vi "FEED_Check_For_indicator.vi"(7 "CURRENT PLAN":refnum<vi>, 8 "error in (no error)":errorcluster) -> (0 "error out":errorcluster)   [LabVIEW 2017]
panel:
  in  "String":string
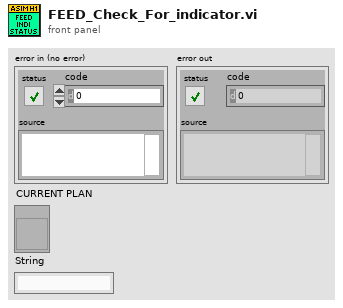
[diagram p1: front panel]
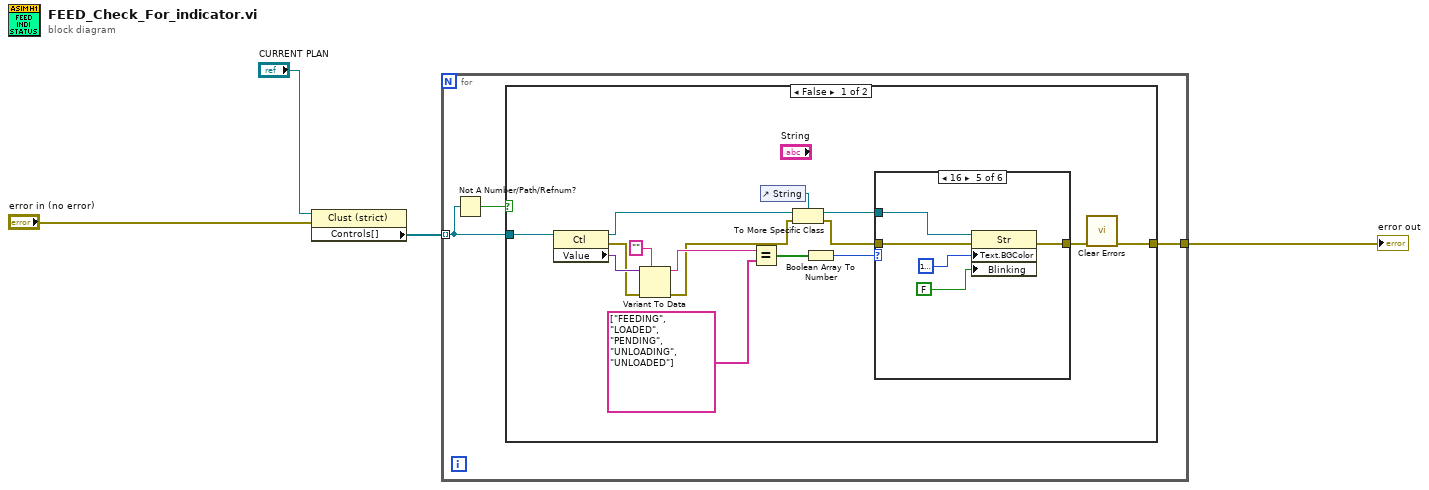
[diagram p0: block diagram]
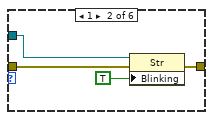
[diagram p3: hidden frame]
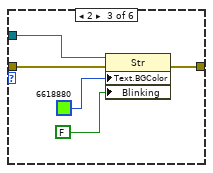
[diagram p4: hidden frame]
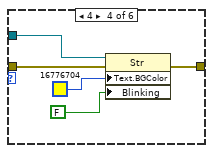
[diagram p5: hidden frame]
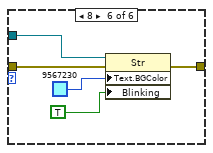
[diagram p6: hidden frame]
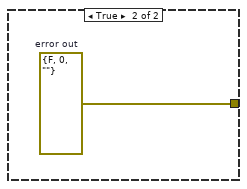
[diagram p7: hidden frame]
diagram:
  n1 = property class="Clust (strict)"(reference="CURRENT PLAN", error in="error in (no error)") -> ("Controls[]"=w2:refnum<vi>[])  [unwired: 2 out]
  n2 = for {
    tunnel: w2 -> [w7] mode=indexing
    tunnel: [w5] -> w4
    n3 = Not A Number/Path/Refnum?(number/path/refnum=w7) -> (NaN/Path/Refnum?=w6:bool)
    n4 = case shown="False" w6 {
      tunnel: w7 -> [w21 _]
      tunnel: [w14 w48] -> w5
      frame False {
        n5 = property class="Ctl"(reference=w21) -> (reference out=w20:refnum<vi>, error out=w16:errorcluster, "Value"=w19:variant)  [unwired: 1 in]
        n6 = Variant To Data(error in=w16, type="", Variant=w19) -> (data=w17:string, error out=w9:errorcluster)
        n7 = Equal?(x=w17, y=string[] ["FEEDING", "LOADED", "PENDING", "UNLOADING", "UNLOADED"]) -> (x = y?=w12:bool[])
        n8 = control-ref of="String"() -> (w11:refnum<vi>)
        n9 = To More Specific Class(target class=w11, reference=w20, error in=w9) -> (specific class reference=w10:refnum<vi>, error out=w8:errorcluster)
        n10 = Boolean Array To Number(Boolean array=w12) -> (number=w13:u32)
        n11 = case shown="16" w13 {
          tunnel: w8 -> [w23 w27 w32 w37 w42 w47]
          tunnel: [w23 w26 w31 w36 w41 w46] -> w15
          tunnel: w10 -> [_ w24 w29 w34 w39 w44]
          frame 0, Default {
          }
          frame 1 {
            n12 = property class="Str"(reference=w24, error in=w27, "Blinking"=TRUE) -> (error out=w26:errorcluster)  [unwired: 1 out]
          }
          frame 2 {
            n13 = property class="Str"(reference=w29, error in=w32, "Text.BGColor"=u32 6618880, "Blinking"=FALSE) -> (error out=w31:errorcluster)  [unwired: 1 out]
          }
          frame 4 {
            n14 = property class="Str"(reference=w34, error in=w37, "Text.BGColor"=u32 16776704, "Blinking"=FALSE) -> (error out=w36:errorcluster)  [unwired: 1 out]
          }
          frame 16 {
            n15 = property class="Str"(reference=w39, error in=w42, "Text.BGColor"=u32 16777226, "Blinking"=FALSE) -> (error out=w41:errorcluster)  [unwired: 1 out]
          }
          frame 8 {
            n16 = property class="Str"(reference=w44, error in=w47, "Text.BGColor"=u32 9567230, "Blinking"=TRUE) -> (error out=w46:errorcluster)  [unwired: 1 out]
          }
        }
        n17 = call <vilib>:"Clear Errors.vi"("error in (no error)"=w15) -> ("error out"=w14:errorcluster)  [unwired: 5 in, 1 out]
      }
      frame True {
        w48 = errorcluster {"status"=FALSE, "code"=0, "source"=""}  # error out
      }
    }
  }
  "error out" <- w4
